vi "ST example routine ESTOP.vi"() -> ()   [LabVIEW 2009]
panel:
  out "ROUTINE\nDONE":bool
  out "Running":bool
  out "Stopped":bool
  in  "EMERGENCY STOP":bool
  out "MOTORS \nOFF":bool
  out "PERFORMED\nWAIST -0.4 RADIANS":bool
  out "Motor Speed\nSteps/sec":string
  out "CHANGED SPEED\nTO 2000":bool
  out "PERFORMED\nWAIST 0.4 RADIANS":bool
  out "STATUS\nREADY":bool
  # "THIS IS A TEST ROUTINE FOR THE MOTIONS\nFIRST IT WILL INITIALIZE THE ROBOT AND THE CONTROLLER\nTHEN IT WILL EXERCISE A JOINT\nCHANGING SPEED BETWEEN MOVES\nIT THEN WILL DE-ENERGIZE THE MOTORS.\n\nTHE FORMAT OF THE ROUTINE ALLOWS FOR AN EMERGENCY\nSTOP BUTTON, SHOWN BELOW."
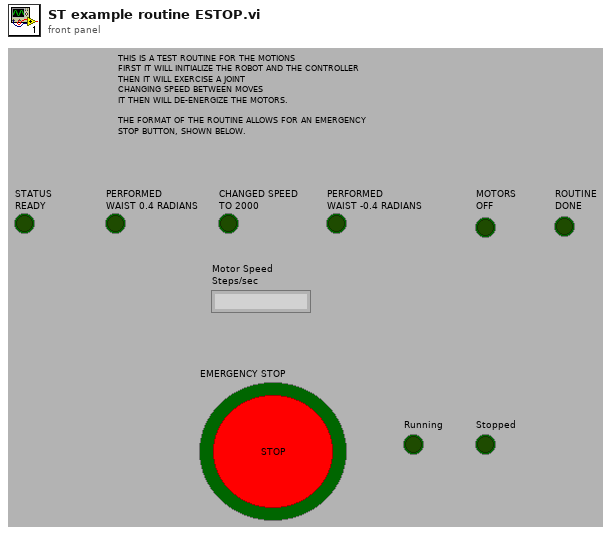
[diagram p1: front panel]
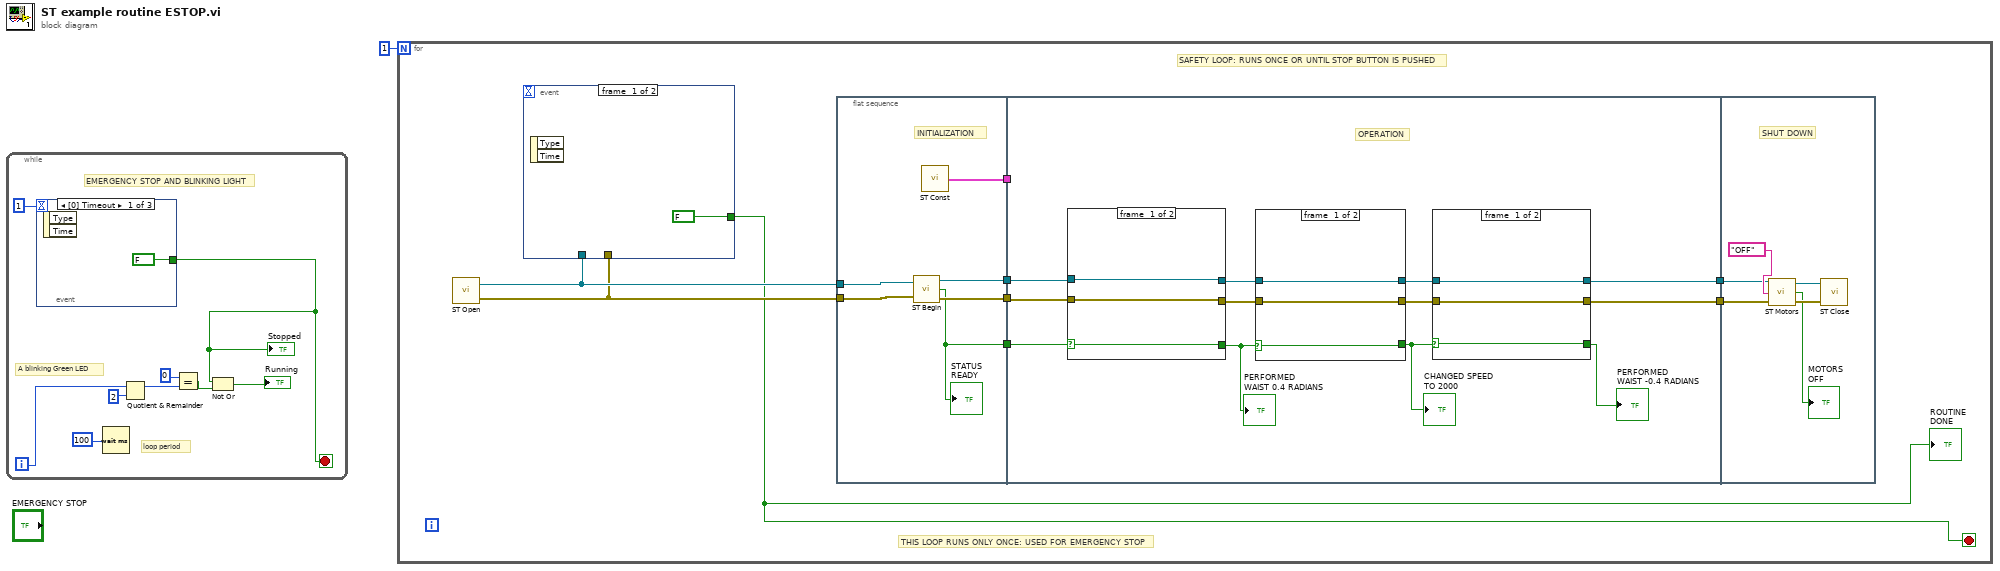
[diagram p0: block diagram]
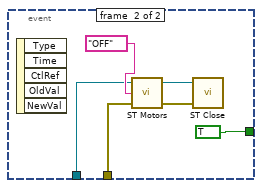
[diagram p2: hidden frame]
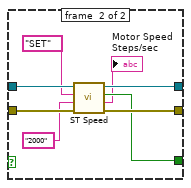
[diagram p3: hidden frame]
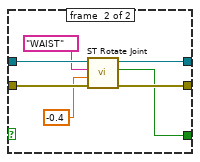
[diagram p4: hidden frame]
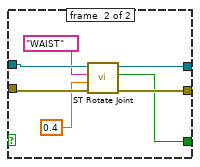
[diagram p5: hidden frame]
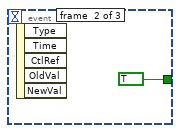
[diagram p6: hidden frame]
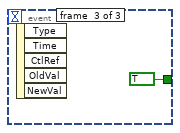
[diagram p7: hidden frame]
diagram:
  n1 = while {
    i -> [w5]
    stop <- w2 stop-if-true
    # "EMERGENCY STOP AND BLINKING LIGHT"
    # "loop period"
    # "A blinking Green LED"
    n2 = event shown="[0] Timeout" {
      selector: _ -> [_ _ _]
      dyn-events: _ -> [_ _ _]
      timeout: 1 -> [_ _ _]
      tunnel: [FALSE TRUE TRUE] -> w2
      event #0 {
        n3 = event-data() -> ()  [unwired: 1 in, 2 out]
      }
      event #1 {
        n4 = event-data() -> ()  [unwired: 1 in, 5 out]
      }
      event #2 {
        n5 = event-data() -> ()  [unwired: 1 in, 5 out]
      }
    }
    "Stopped" <- w2
    n6 = Wait (ms)(milliseconds to wait=u32 100) -> ()  [unwired: 1 out]
    n7 = Quotient & Remainder(x=w5, y=2) -> (x-y*floor(x/y)=w8:i32)  [unwired: 1 out]
    n8 = Equal?(x=0, y=w8) -> (x = y?=w3:bool)
    n9 = Not Or(1:w3, 2:w2) -> (0:→"Running":bool)
  }
  n10 = for {
    N: 1 -> [_]
    stop <- w14 stop-if-true
    # "THIS LOOP RUNS ONLY ONCE: USED FOR EMERGENCY STOP"
    # "SAFETY LOOP: RUNS ONCE OR UNTIL STOP BUTTON IS PUSHED"
    n11 = call "ST Open.vi"() -> ("VISA resource name out"=w16:refnum<visa-resource-name>, "error out"=w15:errorcluster)  [unwired: 1 in]
    n12 = event shown="[1] \"EMERGENCY STOP\": Value Change" {
      selector: _ -> [_ _]
      dyn-events: _ -> [_ _]
      timeout: _ -> [_ _]
      tunnel: [FALSE TRUE] -> w14
      tunnel: w16 -> [_ w26]
      tunnel: w15 -> [_ w25]
      event #0 {
        n13 = event-data() -> ()  [unwired: 1 in, 2 out]
      }
      event #1 {
        n14 = event-data() -> ()  [unwired: 1 in, 5 out]
        n15 = call "ST Motors.vi"("error in (error out)"=w25, "Combo Box"="OFF", "VISA resource name in"=w26) -> ("error out"=w28:errorcluster, "VISA resource name out"=w29:refnum<visa-resource-name>)  [unwired: 1 out]
        n16 = call "ST Close.vi"("error in (no error)"=w28, "VISA resource name"=w29) -> ()
      }
    }
    "ROUTINE\nDONE" <- w14
    n17 = flat-sequence {
      tunnel: [w35] -> w22
      tunnel: [w34] -> w21
      tunnel: [w33] -> w20
      tunnel: [w32] -> w17
      tunnel: w16 -> [w31]
      tunnel: w15 -> [w30]
      tunnel: w22 -> [w41]
      tunnel: w21 -> [w40]
      tunnel: [w38] -> w19
      tunnel: [w37] -> w18
      tunnel: w20 -> [w36]
      tunnel: w17 -> [_]
      tunnel: w19 -> [w81]
      tunnel: w18 -> [w80]
      frame #0 {
        # "INITIALIZATION"
        n18 = call "ST Begin.vi"("VISA resource name in"=w31, "error in"=w30) -> ("VISA resource name out"=w35:refnum<visa-resource-name>, "Begin Complete"=w33:bool, "error out"=w34:errorcluster)
        "STATUS\nREADY" <- w33
        n19 = call "ST Const.vi"() -> ("Robot Constants"=w32:cluster{i32[], i32[], dbl[]})
      }
      frame #1 {
        # "OPERATION"
        n20 = case shown="True" w36 {
          selector: w36 -> [w69 _]
          tunnel: w41 -> [w71 w78]
          tunnel: w40 -> [w70 w77]
          tunnel: [w71 w75] -> w47
          tunnel: [w70 w74] -> w46
          tunnel: [w69 w73] -> w43
          frame #0 {
          }
          frame #1 {
            n21 = call "ST Rotate Joint.vi"("error in (no error)"=w77, "Radians"=0.4, "Joint to rotate"="WAIST" ("JOINT NAME"), "VISA resource name"=w78) -> ("error out"=w74:errorcluster, "Ready and OK"=w73:bool, "VISA resource name out"=w75:refnum<visa-resource-name>)  [unwired: 2 out]
          }
        }
        "PERFORMED\nWAIST 0.4 RADIANS" <- w43
        n22 = case shown="True" w43 {
          selector: w43 -> [w48 _]
          tunnel: w47 -> [w50 w58]
          tunnel: w46 -> [w49 w57]
          tunnel: [w49 w56] -> w45
          tunnel: [w50 w55] -> w44
          tunnel: [w48 w52] -> w42
          frame #0 {
          }
          frame #1 {
            n23 = call "ST Speed.vi"("error in (error out)"=w57, "New Speed"="2000", "Action"="SET", "VISA resource name in"=w58) -> ("error out"=w56:errorcluster, "Motor Speed"=→"Motor Speed\nSteps/sec":string, "Complete"=w52:bool, "VISA resource name out"=w55:refnum<visa-resource-name>)
          }
        }
        "CHANGED SPEED\nTO 2000" <- w42
        n24 = case shown="True" w42 {
          selector: w42 -> [w59 _]
          tunnel: w44 -> [w61 w68]
          tunnel: w45 -> [w60 w67]
          tunnel: [w61 w65] -> w38
          tunnel: [w60 w64] -> w37
          tunnel: [w59 w63] -> w39
          frame #0 {
          }
          frame #1 {
            n25 = call "ST Rotate Joint.vi"("error in (no error)"=w67, "Radians"=-0.4, "Joint to rotate"="WAIST" ("JOINT NAME"), "VISA resource name"=w68) -> ("error out"=w64:errorcluster, "Ready and OK"=w63:bool, "VISA resource name out"=w65:refnum<visa-resource-name>)  [unwired: 2 out]
          }
        }
        "PERFORMED\nWAIST -0.4 RADIANS" <- w39
      }
      frame #2 {
        # "SHUT DOWN"
        n26 = call "ST Motors.vi"("error in (error out)"=w80, "Combo Box"="OFF", "VISA resource name in"=w81) -> ("error out"=w83:errorcluster, "SESSION \nENDED"=→"MOTORS \nOFF":bool, "VISA resource name out"=w84:refnum<visa-resource-name>)
        n27 = call "ST Close.vi"("error in (no error)"=w83, "VISA resource name"=w84) -> ()
      }
    }
  }
